vi "LV_ATS.vi"(5 "test json in":string) -> (0 "formatted test json out":string, 1 "ats json out":string, 2 "PASS":bool, 3 "error out":errorcluster)   [LabVIEW 2019]
panel:
  out "error out 2":errorcluster
  in  "ats json in":string
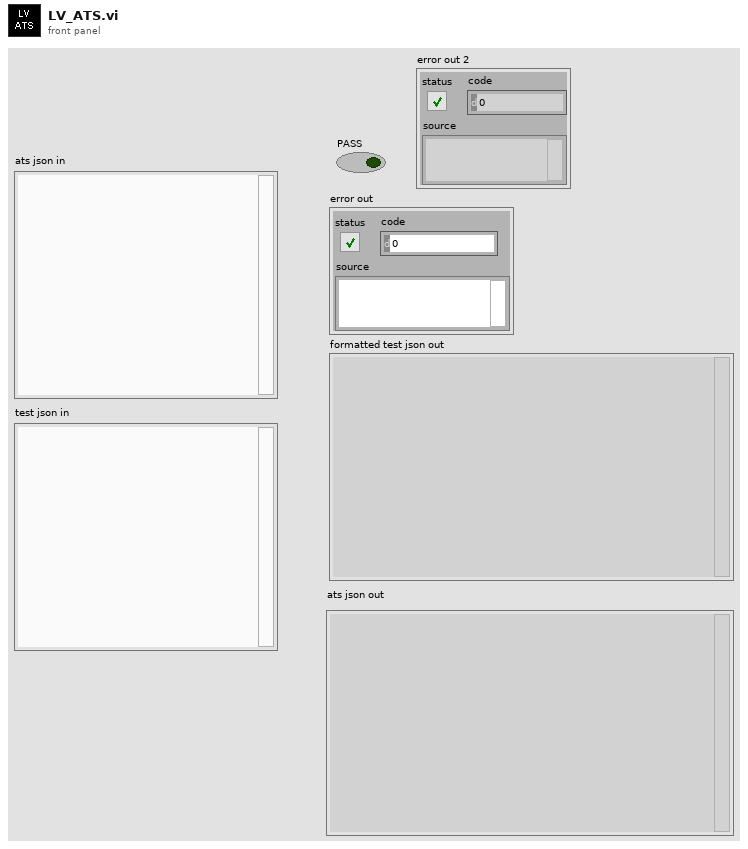
[diagram p1: front panel]
types:
  T1 = enum16{"open", "replace", "create", "open or create", "replace or create", "replace or create with confirmation"}
  T2 = cluster{"description":string, "error type":enum32{"generic failure", "boundary case", "precision", "expected error"}}[]
  T3 = cluster{"control\nname":string, "type\ndescriptor":i16[], "flattened\ndata":string}[]
  T4 = cluster{"Load time (ms)":u32, "DataSize after execution":u32, "Execute time":u32, "DataSize before execution":u32}
  T5 = cluster{"array of error description":cluster{"description":string, "error type":string}[], "outputs":cluster{"control\nname":string, "type\ndescriptor":i16[], "flattened\ndata":string}[], "error out 2":errorcluster, "Metrics":cluster{"Load time (ms)":u32, "DataSize after execution":u32, "Execute time":u32, "DataSize before execution":u32}, "array output?":bool}
  T6 = cluster{"description":string, "error type":string}[]
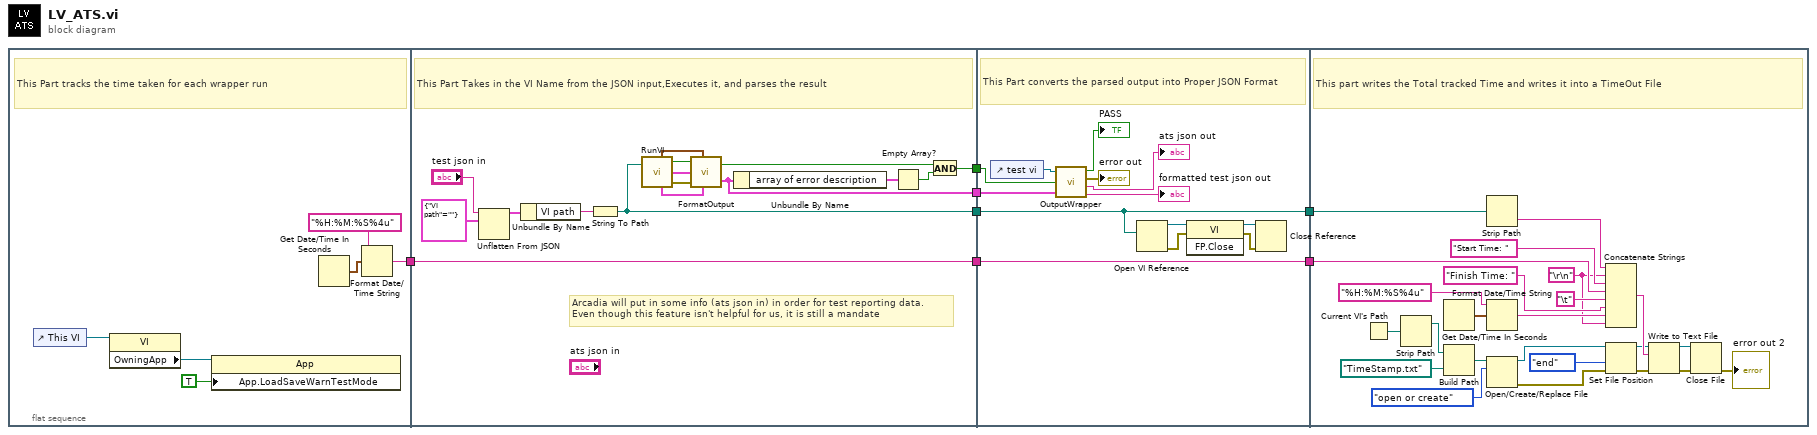
[diagram p0: block diagram]
diagram:
  n1 = flat-sequence {
    tunnel: [w11] -> w5
    tunnel: [w23] -> w7
    tunnel: [w26] -> w6
    tunnel: w5 -> [w20]
    tunnel: [w20] -> w4
    tunnel: [w19] -> w2
    tunnel: w7 -> [w40]
    tunnel: w6 -> [w41]
    tunnel: w4 -> [w35]
    tunnel: [w35] -> w3
    tunnel: w2 -> [w34]
    tunnel: [w34] -> w1
    tunnel: w3 -> [w47]
    tunnel: w1 -> [w57]
    frame #0 {
      # "This Part tracks the time taken for each wrapper run"
      n2 = control-ref of="This VI"() -> (w10:refnum<vi>)
      n3 = property class="VI"(reference=w10) -> ("OwningApp"=w9:refnum<vi>)  [unwired: 1 in, 2 out]
      n4 = property class="App"(reference=w9, "App.LoadSaveWarnTestMode"=TRUE ("Load and Save Warnings:Auto Test Mode")) -> ()  [unwired: 1 in, 2 out]
      n5 = Get Date/Time In Seconds() -> (seconds since 1Jan1904=w13:timestamp)
      n6 = Format Date/Time String(time format string (%c)="%H:%M:%S%4u", seconds (now)=w13) -> (date/time string=w11:string)  [unwired: 1 in]
    }
    frame #1 {
      # "Arcadia will put in some info (ats json in) in order for test reporting data.\nEven though this feature isn't helpful for us, it is still a mandate"
      # "This Part Takes in the VI Name from the JSON input,Executes it, and parses the result"
      n7 = Unflatten From JSON(JSON string="test json in", type and defaults=cluster{"VI path":string} {"VI path"=""}) -> (value=w27:cluster{"VI path":string})  [unwired: 5 in, 1 out]
      n8 = Unbundle By Name(w27) -> ("VI path"=w25:string)
      n9 = String To Path(string=w25) -> (path=w19:path)
      n10 = call "RunVI.vi"("VI path"=w19) -> ("error out"=w15:errorcluster, "array of error description"=w14:T2, "outputs"=w16:T3, "array output?"=w17:bool, "Metrics"=w18:T4)  [unwired: 1 in]
      n11 = call "FormatOutput.vi"("array output?"=w17, "Metrics"=w18, "outputs"=w16, "error out 2"=w15, "array of error description"=w14) -> ("Pass"=w24:bool, "FinalCluster"=w23:T5)
      n12 = Unbundle By Name(w23) -> ("array of error description"=w22:T6)
      n13 = Empty Array?(array=w22) -> (empty?=w21:bool)
      n14 = And(x=w24, y=w21) -> (x .and. y?=w26:bool)
    }
    frame #2 {
      # "This Part converts the parsed output into Proper JSON Format"
      n15 = control-ref of="test vi"() -> (w42:refnum<vi>)
      n16 = call "OutputWrapper.vi"("VI in"=w42, "pass"=w41, "FinalCluster"=w40) -> ("PASS"=→"PASS":bool, "error out"=→"error out":errorcluster, "ats json out"=→"ats json out":string, "formatted test json out"=→"formatted test json out":string)
      n17 = Open VI Reference(vi path=w34) -> (vi reference=w33:refnum<vi>, error out=w32:errorcluster)  [unwired: 5 in]
      n18 = invoke class="VI" method="FP.Close"(reference=w33, error in=w32) -> (reference out=w30:refnum<vi>, error out=w31:errorcluster)  [unwired: 1 in, 1 out]
      n19 = Close Reference(reference=w30, error in (no error)=w31) -> ()  [unwired: 1 out]
    }
    frame #3 {
      w43 = "\r\n"
      # "This part writes the Total tracked Time and writes it into a TimeOut File"
      n20 = Current VI's Path() -> (path=w55:path)
      n21 = Strip Path(path=w55) -> (stripped path=w54:path)  [unwired: 1 out]
      n22 = Get Date/Time In Seconds() -> (seconds since 1Jan1904=w65:timestamp)
      n23 = Build Path(base path=w54, name or relative path=path "TimeStamp.txt") -> (appended path=w58:path)
      n24 = Strip Path(path=w57) -> (name=w56:string)  [unwired: 1 out]
      n25 = Format Date/Time String(time format string (%c)="%H:%M:%S%4u", seconds (now)=w65) -> (date/time string=w44:string)  [unwired: 1 in]
      n26 = Open/Create/Replace File(file path (use dialog)=w58, operation (0:open)=T1."open or create") -> (refnum out=w53:refnum<file>, error out=w52:errorcluster)  [unwired: 4 in, 1 out]
      n27 = Concatenate Strings(w56, w43, "Start Time: " ("string"), w47, "\t", "Finish Time: " ("string"), w44, w43) -> (w63:string)
      n28 = Set File Position(refnum=w53, from (0:start)=enum16{"start", "end", "current"}."end", error in=w52) -> (refnum out=w50:refnum<file>, error out=w49:errorcluster)  [unwired: 1 in]
      n29 = Write to Text File(file (use dialog)=w50, text=w63, error in=w49) -> (refnum out=w62:refnum<file>, error out=w61:errorcluster)  [unwired: 1 in, 1 out]
      n30 = Close File(refnum=w62, error in=w61) -> (error out=→"error out 2":errorcluster)  [unwired: 1 out]
    }
  }
